vi "FTW-Publisher-Construct.vi"(5 "Address":string, 7 "Identity":string, 11 "error in":errorcluster, 12 "Send Buffer Depth (1)":i32=1, 13 "Send Timeout (-1)":i32=-1) -> (4 "FTW-Publisher Out":refnum<class "FTW-Publisher.lvclass">, 6 "Actual Address":string, 15 "error out":errorcluster)   [LabVIEW 2013, in "FTW-Publisher.lvclass"]
uses:
  FTW-Publisher.lvclass
  Package/Base/FTW-Package.lvclass
  FTW-Publisher.lvclass/FTW-Publisher.ctl
  Ether/FTW-Ether-EndpointType.ctl
  Endpoint/FTW-Endpoint.lvclass
  Ether/FTW-Ether.lvclass
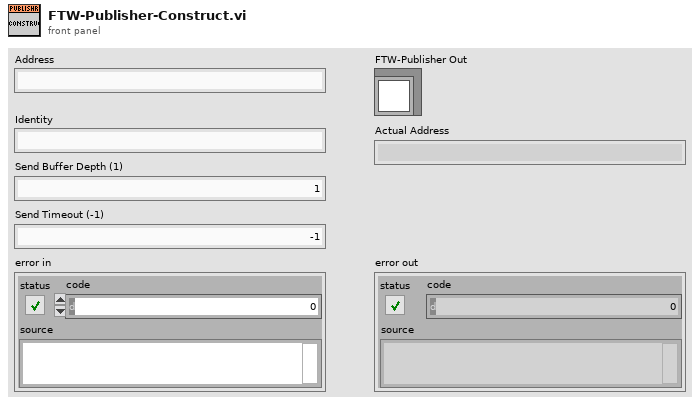
[diagram p1: front panel]
types:
  T1 = typedef "FTW-Ether.lvclass/FTW-Ether-EndpointType.ctl" = enum16{"Server", "Client", "Publisher", "Subscriber"}
  T2 = typedef "FTW-Ether.lvclass/FTW-Ether-MessageTransportScheme.ctl" = enum16{"In process (inproc://)", "TCP (tcp://)"}
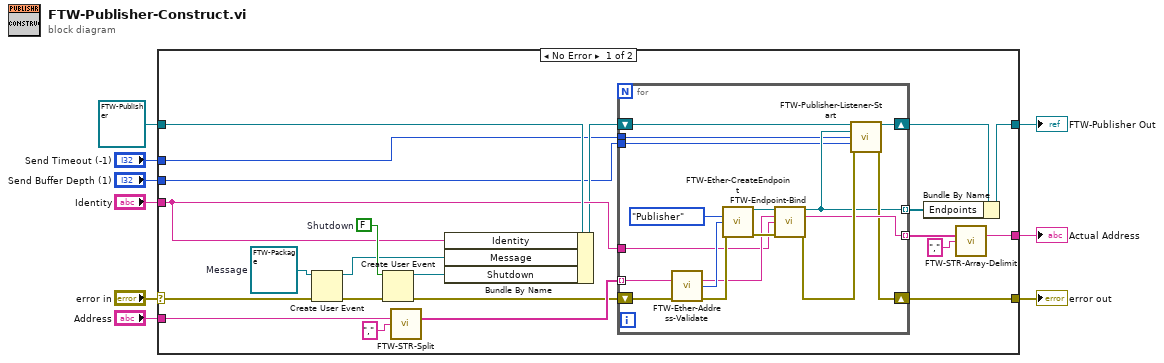
[diagram p0: block diagram]
diagram:
  n1 = case shown="No Error" "error in" {
    selector: "error in" -> [w19 w50]
    tunnel: [w14 w50] -> w8
    tunnel: [w28 w49] -> w7
    tunnel: "Address" -> [w21 _]
    tunnel: [w24 _] -> w5
    tunnel: "Identity" -> [w17 _]
    tunnel: "Send Timeout (-1)" -> [w11 _]
    tunnel: "Send Buffer Depth (1)" -> [w10 _]
    tunnel: refnum<class "FTW-Publisher.lvclass"> refnum ("LVmsg_Router.lvclass") -> [w27 w49]
    frame No Error {
      w29 = FALSE  # Shutdown
      w31 = refnum<class "FTW-Package.lvclass"> refnum  # Message
      n2 = Create User Event(user event datatype=w31, error in=w19) -> (user event=w16:refnum<user-event>, error out=w30:errorcluster)
      n3 = Create User Event(user event datatype=w29, error in=w30) -> (user event=w15:refnum<user-event>, error out=w18:errorcluster)
      n4 = call "FTW-STR-Split.vi"("Delimited String"=w21, "Delimiter"="," ("Delimited String")) -> ("Array of Strings"=w23:string[])  [unwired: 13 in]
      n5 = Bundle By Name(cluster=w27, "Identity"=w17, "Message"=w16, "Shutdown"=w15) -> (w13:refnum<class "FTW-Publisher.lvclass">)
      n6 = for {
        tunnel: w23 -> [w48] mode=indexing
        tunnel: [w34] -> w26 mode=indexing
        tunnel: w17 -> [w39]
        tunnel: [w38] -> w25 mode=indexing
        shift-right: [w37] -> w14
        shift-left: w18 -> [w45]
        shift-right: [w35] -> w12
        shift-left: w13 -> [w36]
        tunnel: w11 -> [w33]
        tunnel: w10 -> [w32]
        n7 = call "FTW-Ether-Address-Validate.vi"("Address"=w48, "error in"=w45) -> ("Sanitized Address"=w40:string, "Message Transport Scheme"=w47:T2, "error out"=w46:errorcluster)  [unwired: 11 in]
        n8 = call "FTW-Ether-CreateEndpoint.vi"("Endpoint Type"=FTW-Ether-EndpointType."Publisher", "Message Transport Scheme"=w47, "error in"=w46) -> ("FTW Endpoint"=w41:refnum<class "FTW-Endpoint.lvclass">, "error out"=w43:errorcluster)  [unwired: 11 in]
        n9 = call-dynamic "FTW-Endpoint-Bind.vi"("FTW Endpoint"=w41, "Endpoint Address"=w40, "Requested Identity"=w39, "error in"=w43) -> ("FTW Endpoint out"=w34:refnum<class "FTW-Endpoint.lvclass">, "Actual Endpoint Address"=w38:string, "error out"=w42:errorcluster)  [unwired: 8 in, 1 out]
        n10 = call "FTW-Publisher-Listener-Start.vi"("FTW Publisher In"=w36, "FTW Endpoint"=w34, "Send Timeout"=w33, "Send Buffer Depth"=w32, "error in"=w42) -> ("FTW Publisher Out"=w35:refnum<class "FTW-Publisher.lvclass">, "error out"=w37:errorcluster)  [unwired: 9 in]
      }
      n11 = Bundle By Name(cluster=w12, "Endpoints"=w26) -> (w28:refnum<class "FTW-Publisher.lvclass">)
      n12 = call "FTW-STR-Array-Delimit.vi"("Array of Strings"=w25, "Delimiter"="," ("Delimited String")) -> ("Delimited String"=w24:string)  [unwired: 13 in]
    }
    frame Error {
    }
  }
  "FTW-Publisher Out" <- w7
  "error out" <- w8
  "Actual Address" <- w5
